vi "open door.vi"(7 "input":i32) -> (4 "1":u16(ring), 6 "2":u16(ring), 8 "3":u16(ring), 10 "4":u16(ring), 15 "5":u16(ring))   [LabVIEW 2020]
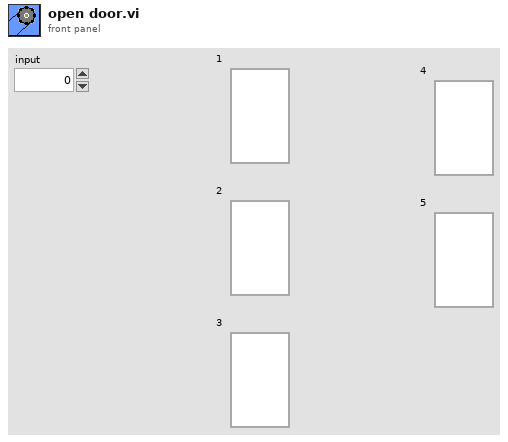
[diagram p1: front panel]
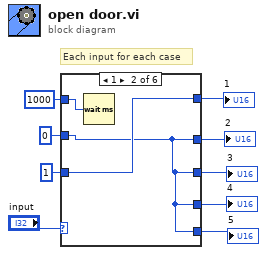
[diagram p0: block diagram]
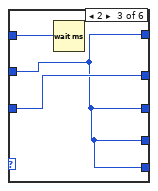
[diagram p3: hidden frame]
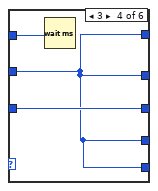
[diagram p4: hidden frame]
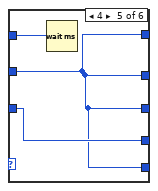
[diagram p5: hidden frame]
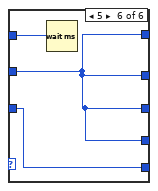
[diagram p6: hidden frame]
diagram:
  # "Each input for each case"
  n1 = case shown="1" "input" {
    tunnel: u32 1000 ("milliseconds to wait") -> [_ w11 w16 w19 w22 w25]
    tunnel: u16 1 ("1") -> [_ w13 w15 w18 w21 w24]
    tunnel: [w10 w12 w14 w17 w20 w24] -> w4
    tunnel: [w10 w13 w14 w17 w20 w23] -> w9
    tunnel: [w10 w12 w14 w17 w21 w23] -> w5
    tunnel: [w10 w12 w15 w17 w20 w23] -> w6
    tunnel: [w10 w12 w14 w18 w20 w23] -> w7
    tunnel: u16 0 ("1") -> [w10 w12 w14 w17 w20 w23]
    frame 0, Default {
    }
    frame 1 {
      n2 = Wait (ms)(milliseconds to wait=w11) -> ()  [unwired: 1 out]
    }
    frame 2 {
      n3 = Wait (ms)(milliseconds to wait=w16) -> ()  [unwired: 1 out]
    }
    frame 3 {
      n4 = Wait (ms)(milliseconds to wait=w19) -> ()  [unwired: 1 out]
    }
    frame 4 {
      n5 = Wait (ms)(milliseconds to wait=w22) -> ()  [unwired: 1 out]
    }
    frame 5 {
      n6 = Wait (ms)(milliseconds to wait=w25) -> ()  [unwired: 1 out]
    }
  }
  "5" <- w4
  "1" <- w9
  "2" <- w6
  "3" <- w7
  "4" <- w5
